vi "rqcBob Train Config.vi"(0 "rqcBob in":refnum<class "rqcBob.lvclass">, 1 "Train.Generation Mode":T1=enum."train sequence.single", 5 "Train.Period":u16=4000, 7 "Train.Number of Pulses":u16=1, 9 "Train.Number of Trains":u16=4000, 11 "error in (no error)":errorcluster, 12 "Train.First Pulse Delay Mode":T2=enum."every train", 13 "Train.First Pulse Delay":u16=55) -> (4 "rqcBob out":refnum<class "rqcBob.lvclass">, 15 "error out":errorcluster)   [LabVIEW 2018, in "rqcBob.lvclass"]
uses:
  rqcBob.lvclass
  FPGA/rqcBob/Custom Controls/Pulse Train/rqcBob Pulse Train.First Pulse Delay Mode.ctl
  FPGA/rqcBob/Custom Controls/Pulse Train/rqcBob Pulse Train.Generation Mode.ctl
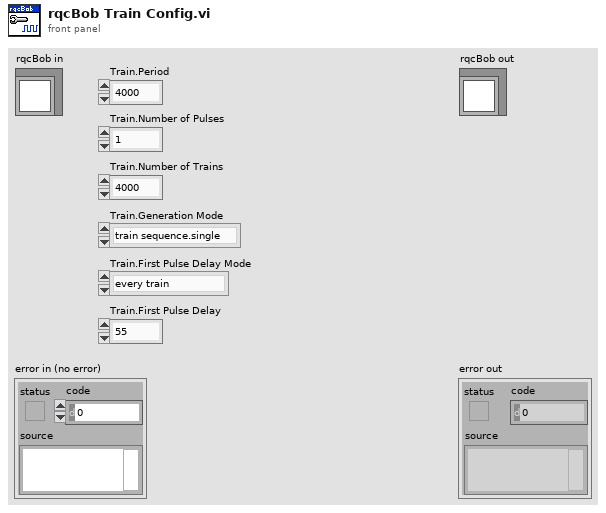
[diagram p1: front panel]
types:
  T1 = typedef "rqcBob Pulse Train.Generation Mode.ctl" = enum8{"single train", "train sequence.single", "train sequence.wait for trigger", "continuous"}
  T2 = typedef "rqcBob Pulse Train.First Pulse Delay Mode.ctl" = enum8{"none", "every train", "first train"}
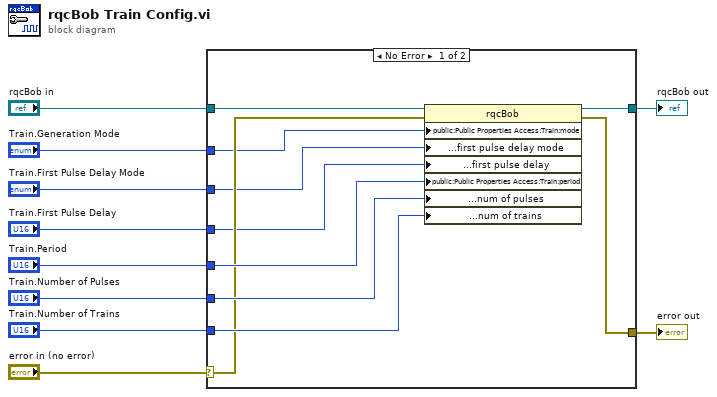
[diagram p0: block diagram]
diagram:
  n1 = case shown="No Error" "error in (no error)" {
    selector: "error in (no error)" -> [w14 w22]
    tunnel: [w19 w22] -> w9
    tunnel: [w20 w21] -> w7
    tunnel: "rqcBob in" -> [w15 w21]
    tunnel: "Train.Period" -> [w18 _]
    tunnel: "Train.Number of Pulses" -> [w17 _]
    tunnel: "Train.Number of Trains" -> [w16 _]
    tunnel: "Train.Generation Mode" -> [w13 _]
    tunnel: "Train.First Pulse Delay Mode" -> [w12 _]
    tunnel: "Train.First Pulse Delay" -> [w11 _]
    frame No Error {
      n2 = property class="rqcBob"(reference=w15, error in=w14, "public:Public Properties Access:Train:mode"=w13, "public:Public Properties Access:Train:first pulse delay mode"=w12, "public:Public Properties Access:Train:first pulse delay"=w11, "public:Public Properties Access:Train:period"=w18, "public:Public Properties Access:Train:num of pulses"=w17, "public:Public Properties Access:Train:num of trains"=w16) -> (reference out=w20:refnum<class "rqcBob.lvclass">, error out=w19:errorcluster)
    }
    frame Error {
    }
  }
  "error out" <- w9
  "rqcBob out" <- w7
